vi "cluster_v15.vi"() -> ()   [LabVIEW 2009]
panel:
  in  "stop":bool
  in  "Numarul afisat pe prima coloana":i16(slide) scale=0.0..255.0
  out "Digital Waveform Graph":T1(graph)
  # "Forma de unda pentru un numarator pe 8 biti"
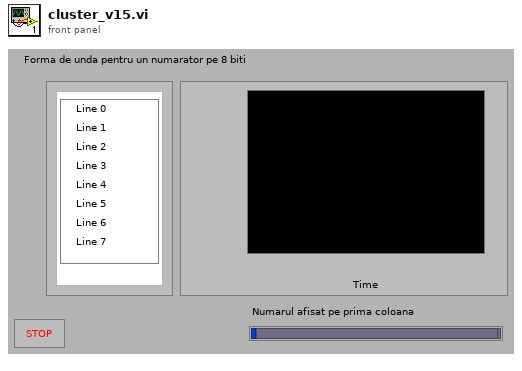
[diagram p1: front panel]
types:
  T1 = cluster{i32, "Latimea unei pozitii":i32, u8[], "Numarul de octeti luati impreuna":i32}
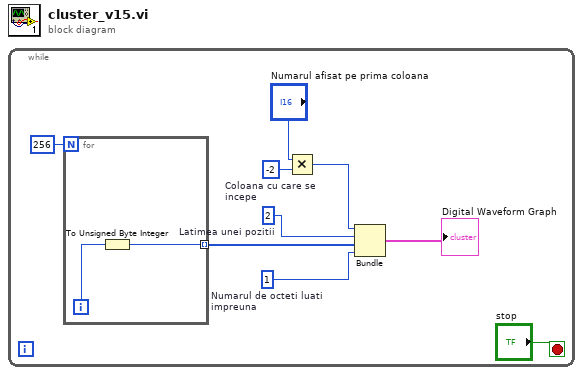
[diagram p0: block diagram]
diagram:
  n1 = while {
    stop <- "stop" stop-if-true
    w5 = 2  # Latimea unei pozitii
    w6 = -2  # Coloana cu care se incepe
    w7 = 1  # Numarul de octeti luati impreuna
    n2 = for {
      N: 256 -> [_]
      tunnel: [w10] -> w9 mode=indexing
      i -> [w11]
      n3 = To Unsigned Byte Integer(number=w11) -> (unsigned 8bit integer=w10:u8)
    }
    n4 = Multiply(x="Numarul afisat pe prima coloana", y=w6) -> (x*y=w3:i32)
    n5 = Bundle(w3, "Latimea unei pozitii"=w5, w9, "Numarul de octeti luati impreuna"=w7) -> (→"Digital Waveform Graph":T1)  [unwired: 1 in]
  }
